vi "digitally_ros_joystick.vi"() -> ()   [LabVIEW 2019]
uses:
  <vilib>/addons/eal4LabVIEW/ApiLib/Connection control/ealApiConnect_string.vi
  <vilib>/Utility/inputDevices.llb/joystickAcquire.vi
  <vilib>/Utility/inputDevices.llb/closeJoystick.vi
  <vilib>/addons/eal4LabVIEW/eal4LabVIEW.lvlib
panel:
  out "I value":i32
  out "Y axis 2":i32
  out "Y axis":i32
  out "X axis":i32
  out "error out":errorcluster
  out "Is joystick used?":bool
  out "Is manual control on?":bool
  out "RPM 3 Joystick":dbl
  out "RPM 1 Joystick":dbl
  out "RPM 2 Joystick":dbl
  out "Is joystick used?":bool[](array[boolean])
  in  "Activate manual control":bool
  out "Is the PID fnished?":bool[](array[boolean])
  out "In Range? (1)":bool
  out "In Range? (2)":bool
  out "In Range? (3)":bool
  in  "condition 6":i32(ring) items=["AXIS_CONDITION_ACTIVE"=0, "AXIS_CONDITION_PARKING"=1, "AXIS_CONDITION_DEACTIVATED"=2, "AXIS_CONDITION_ACTIVE_DECOUPLED"=4, "AXIS_CONDITION_PARKING_DECOUPLED"=5, "AXIS_CONDITION_DEACTIVATED_DECOUPLED"=6, "AXIS_CONDITION_ACTIVE_PARAMETERIZATION"=8, "AXIS_CONDITION_PARKING_PARAMETERIZATION"=9, "AXIS_CONDITION_DEACTIVATED_PARAMETERIZATION"=10, "AXIS_CONDITION_ACTIVE_DECOUPLED_PARAMETERIZATION"=12, "AXIS_CONDITION_PARKING_DECOUPLED_PARAMETERIZATION"=13, "AXIS_CONDITION_DEACTIVATED_DECOUPLED_PARAMETERIZATION"=14]
  in  "slave index 6":i32
  in  "condition 5":i32(ring) items=["AXIS_CONDITION_ACTIVE"=0, "AXIS_CONDITION_PARKING"=1, "AXIS_CONDITION_DEACTIVATED"=2, "AXIS_CONDITION_ACTIVE_DECOUPLED"=4, "AXIS_CONDITION_PARKING_DECOUPLED"=5, "AXIS_CONDITION_DEACTIVATED_DECOUPLED"=6, "AXIS_CONDITION_ACTIVE_PARAMETERIZATION"=8, "AXIS_CONDITION_PARKING_PARAMETERIZATION"=9, "AXIS_CONDITION_DEACTIVATED_PARAMETERIZATION"=10, "AXIS_CONDITION_ACTIVE_DECOUPLED_PARAMETERIZATION"=12, "AXIS_CONDITION_PARKING_DECOUPLED_PARAMETERIZATION"=13, "AXIS_CONDITION_DEACTIVATED_DECOUPLED_PARAMETERIZATION"=14]
  in  "slave index 5":i32
  in  "condition 4":i32(ring) items=["AXIS_CONDITION_ACTIVE"=0, "AXIS_CONDITION_PARKING"=1, "AXIS_CONDITION_DEACTIVATED"=2, "AXIS_CONDITION_ACTIVE_DECOUPLED"=4, "AXIS_CONDITION_PARKING_DECOUPLED"=5, "AXIS_CONDITION_DEACTIVATED_DECOUPLED"=6, "AXIS_CONDITION_ACTIVE_PARAMETERIZATION"=8, "AXIS_CONDITION_PARKING_PARAMETERIZATION"=9, "AXIS_CONDITION_DEACTIVATED_PARAMETERIZATION"=10, "AXIS_CONDITION_ACTIVE_DECOUPLED_PARAMETERIZATION"=12, "AXIS_CONDITION_PARKING_DECOUPLED_PARAMETERIZATION"=13, "AXIS_CONDITION_DEACTIVATED_DECOUPLED_PARAMETERIZATION"=14]
  in  "slave index 4":i32
  out "RPM 1 ROS":dbl
  out "RPM 2 ROS":dbl
  out "RPM 3 ROS":dbl
  in  "stop":bool
  out "Return value":dbl[](array[numeric])
  out "Iteration counter":i32
  # "ROS Control"
  # "Joystick Control"
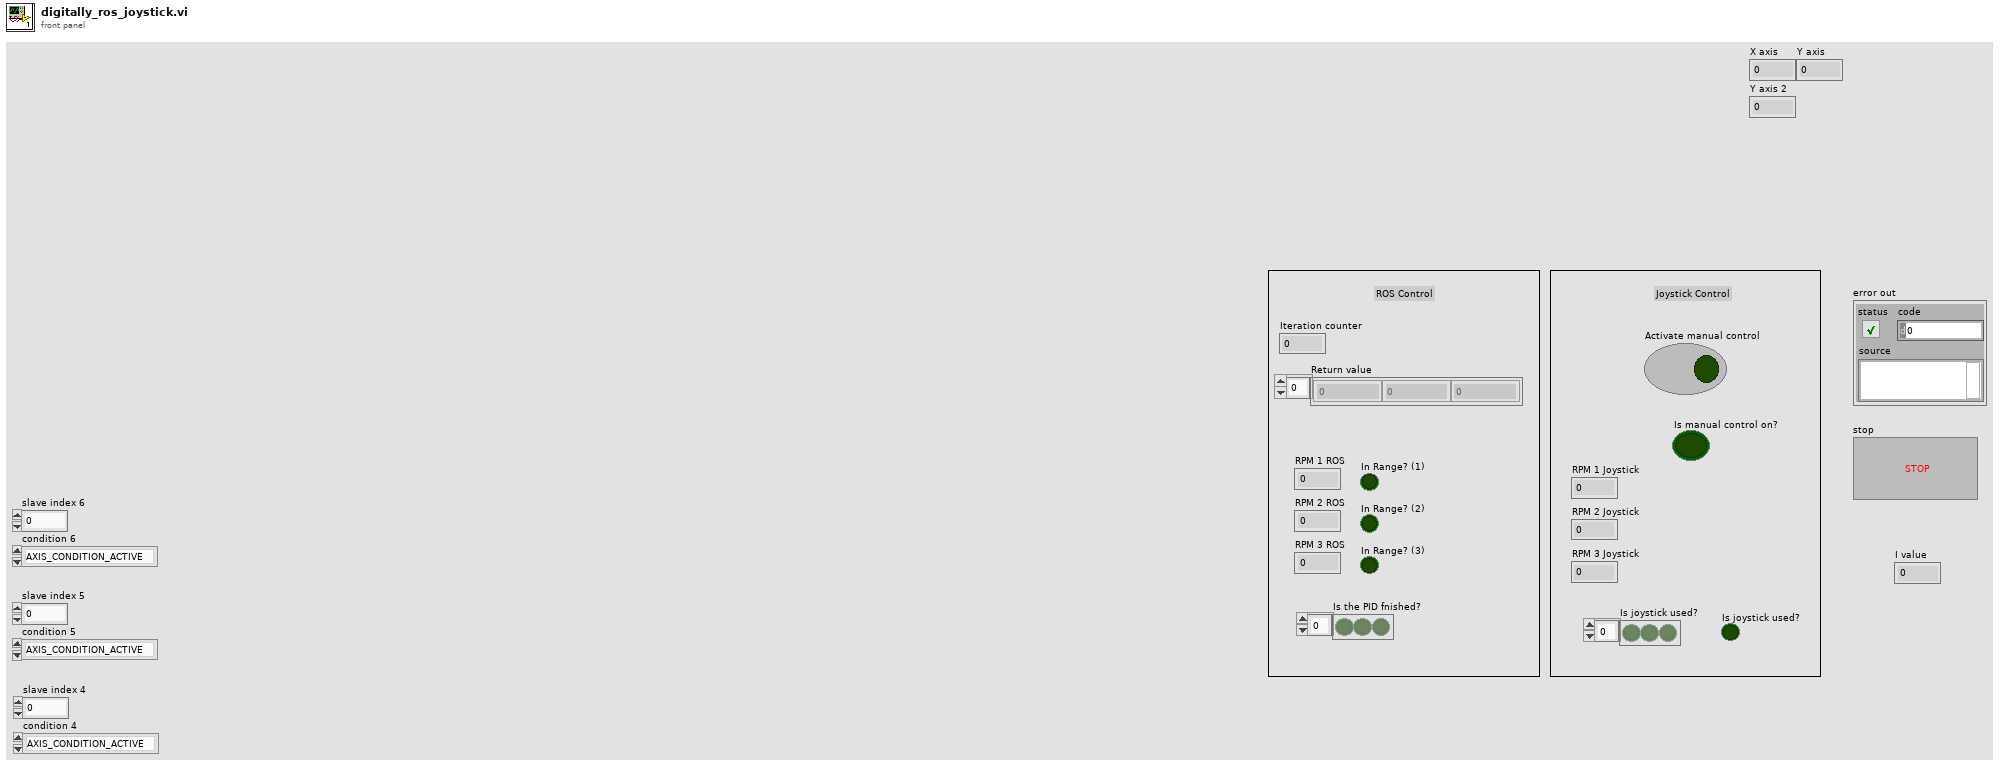
[diagram p1: front panel]
types:
  T1 = cluster{"Velocity":dbl, "Acceleration":dbl, "Deceleration":dbl, "Jerk":dbl}
  T2 = cluster{"X axis":i32, "Y axis":i32, "Z axis":i32, "X axis rotation":i32, "Y axis rotation":i32, "Z axis rotation":i32, "U axis":i32, "V axis":i32}
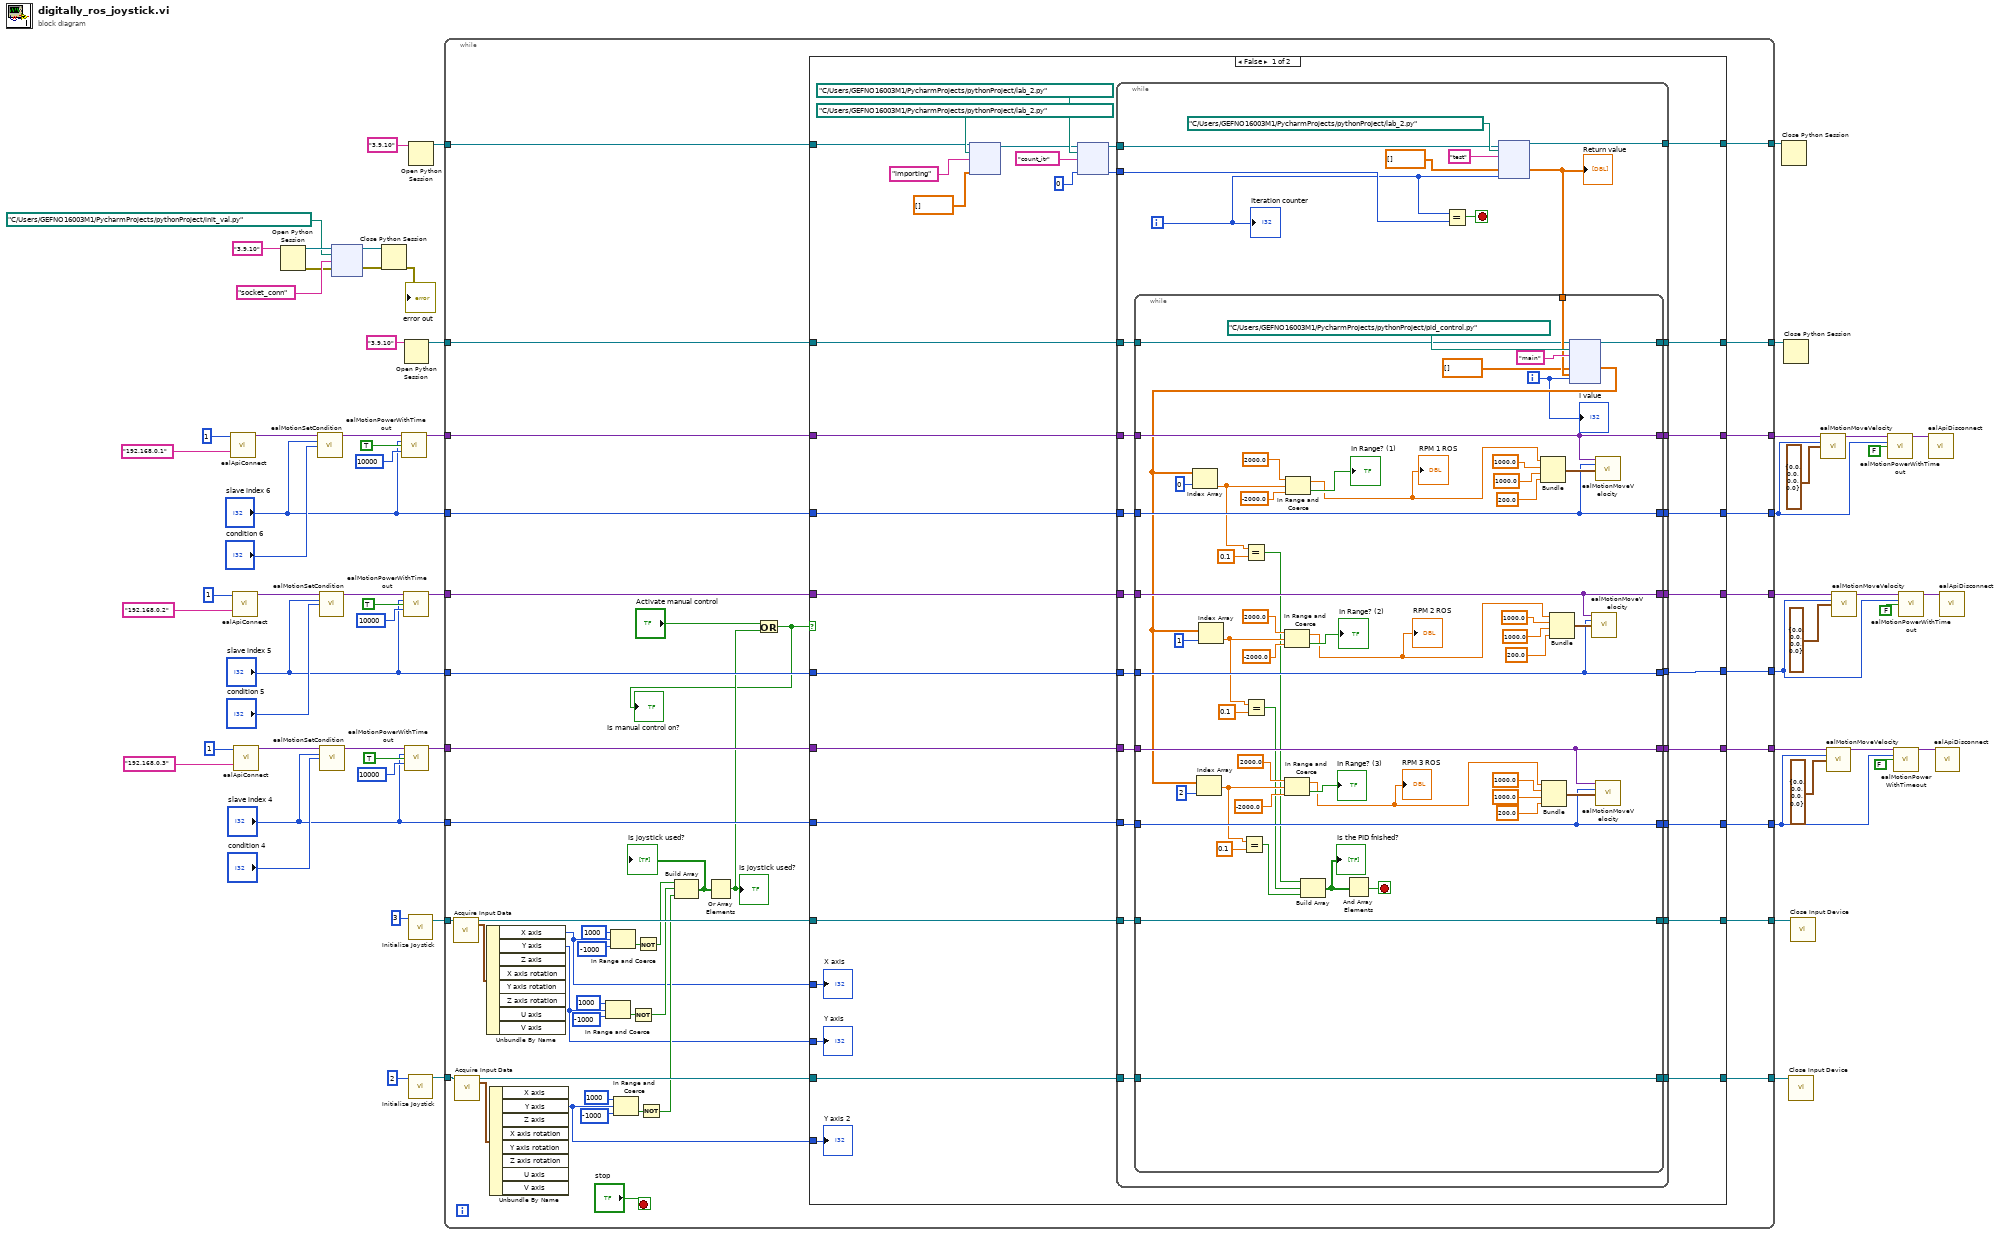
[diagram p0: block diagram]
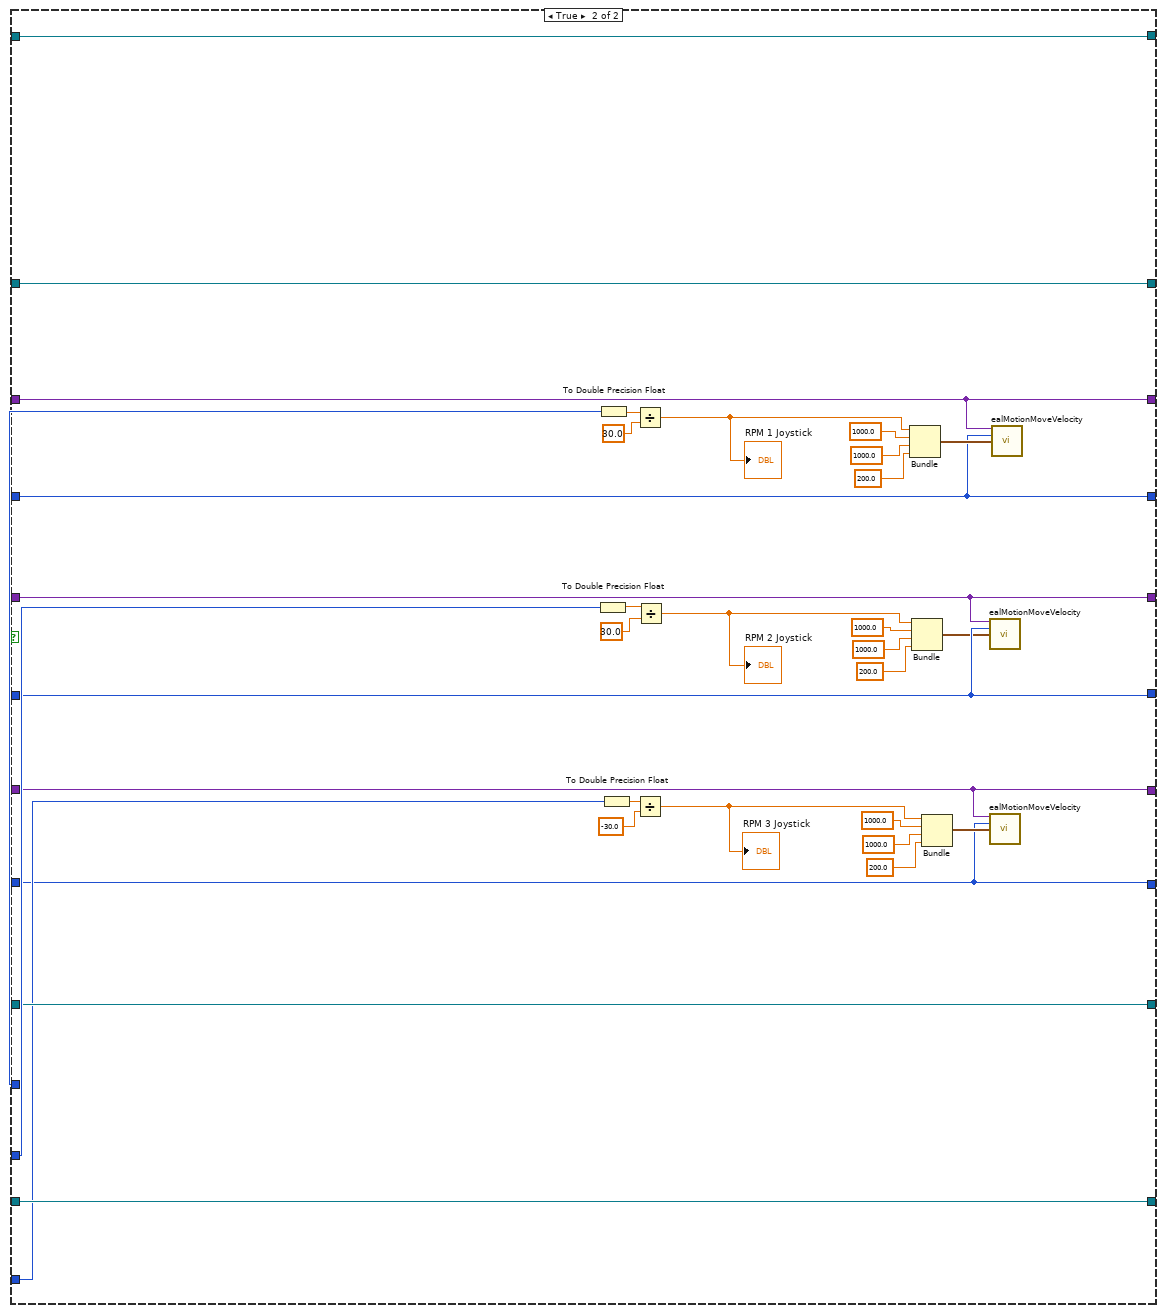
[diagram p2: hidden frame]
diagram:
  n1 = call-poly <vilib>:"ealApiConnect.vi"("maximum no of axes"=1, "ip address"="192.168.0.1") -> ("connection out"=w37:variant)  [unwired: 12 in, 1 out]
  n2 = call-poly <vilib>:"ealApiConnect.vi"("maximum no of axes"=1, "ip address"="192.168.0.2") -> ("connection out"=w44:variant)  [unwired: 12 in, 1 out]
  n3 = call-poly <vilib>:"ealApiConnect.vi"("maximum no of axes"=1, "ip address"="192.168.0.3") -> ("connection out"=w51:variant)  [unwired: 12 in, 1 out]
  n4 = Open Python Session(python version="3.9.10" ("Python version")) -> (session out=w7:refnum<k35>, error out=w3:errorcluster)  [unwired: 2 in]
  n5 = call <vilib>:"ealMotionSetCondition.vi"("connection in"=w37, "slave index"="slave index 6", "condition"="condition 6") -> ("connection out"=w36:variant)  [unwired: 11 in, 1 out]
  n6 = call <vilib>:"ealMotionSetCondition.vi"("connection in"=w44, "slave index"="slave index 5", "condition"="condition 5") -> ("connection out"=w43:variant)  [unwired: 11 in, 1 out]
  n7 = call <vilib>:"ealMotionSetCondition.vi"("connection in"=w51, "slave index"="slave index 4", "condition"="condition 4") -> ("connection out"=w50:variant)  [unwired: 11 in, 1 out]
  n8 = node(w7, path "C:/Users/GEFNO16003M1/PycharmProjects/pythonProject/init_val.py" ("module path"), "socket_conn" ("function name"), w3) -> (w6:refnum<k35>, w2:errorcluster)  [unwired: 2 in, 2 out]
  n9 = Close Python Session(session in=w6, error in=w2) -> (11:→"error out":errorcluster)
  n10 = call <vilib>:"ealMotionPowerWithTimeout.vi"("connection in"=w36, "slave index"="slave index 6", "value"=TRUE, "timeout"=10000) -> ("connection out"=w32:variant)  [unwired: 10 in, 1 out]
  n11 = call <vilib>:"ealMotionPowerWithTimeout.vi"("connection in"=w43, "slave index"="slave index 5", "value"=TRUE, "timeout"=10000) -> ("connection out"=w31:variant)  [unwired: 10 in, 1 out]
  n12 = Open Python Session(python version="3.9.10" ("Python version")) -> (session out=w18:refnum<k35>)  [unwired: 2 in, 1 out]
  n13 = call <vilib>:"ealMotionPowerWithTimeout.vi"("connection in"=w50, "slave index"="slave index 4", "value"=TRUE, "timeout"=10000) -> ("connection out"=w30:variant)  [unwired: 10 in, 1 out]
  n14 = call <vilib>:"Initialize Joystick.vi"("device index"=3) -> ("device ID"=w12:refnum<k1>)  [unwired: 9 in, 1 out]
  n15 = call <vilib>:"Initialize Joystick.vi"("device index"=2) -> ("device ID"=w11:refnum<k1>)  [unwired: 9 in, 1 out]
  n16 = Open Python Session(python version="3.9.10" ("Python version")) -> (session out=w21:refnum<k35>)  [unwired: 2 in, 1 out]
  n17 = while {
    tunnel: w32 -> [w108]
    tunnel: w31 -> [w107]
    tunnel: w30 -> [w106]
    tunnel: [w84] -> w29
    tunnel: [w105] -> w28
    tunnel: "slave index 6" -> [w104]
    tunnel: "slave index 5" -> [w103]
    tunnel: [w102] -> w25
    tunnel: [w96] -> w24
    tunnel: "slave index 4" -> [w101]
    tunnel: w21 -> [w100]
    tunnel: [w99] -> w20
    tunnel: w18 -> [w98]
    tunnel: [w85] -> w17
    tunnel: [w97] -> w16
    tunnel: [w95] -> w15
    tunnel: w12 -> [w92]
    tunnel: w11 -> [w89]
    tunnel: [w94] -> w10
    tunnel: [w93] -> w9
    stop <- "stop" stop-if-true
    n18 = call-poly <vilib>:"Acquire Input Data.vi"("device ID"=w92) -> ("device ID"=w91:refnum<k1>, "axis info"=w90:T2)  [unwired: 14 in, 3 out]
    n19 = call-poly <vilib>:"Acquire Input Data.vi"("device ID"=w89) -> ("device ID"=w88:refnum<k1>, "axis info"=w87:T2)  [unwired: 14 in, 3 out]
    n20 = Unbundle By Name(w90) -> ("X axis"=w68:i32, "Y axis"=w75:i32)  [unwired: 6 out]
    n21 = Unbundle By Name(w87) -> ("Y axis"=w82:i32)  [unwired: 7 out]
    n22 = In Range and Coerce(upper limit=1000, x=w75, lower limit=-1000) -> (In Range?=w77:bool)  [unwired: 1 out]
    n23 = In Range and Coerce(upper limit=1000, x=w68, lower limit=-1000) -> (In Range?=w72:bool)  [unwired: 1 out]
    n24 = In Range and Coerce(upper limit=1000, x=w82, lower limit=-1000) -> (In Range?=w81:bool)  [unwired: 1 out]
    n25 = Not(x=w77) -> (.not. x?=w73:bool)
    n26 = Not(x=w72) -> (.not. x?=w69:bool)
    n27 = Not(x=w81) -> (.not. x?=w80:bool)
    n28 = Build Array(w69, w73, w80) -> (w83:bool[])
    "Is joystick used?" <- w83
    n29 = Or Array Elements(Boolean array=w83) -> (logical OR=w67:bool)
    "Is joystick used?" <- w67
    n30 = Or(x="Activate manual control", y=w67) -> (x .or. y?=w66:bool)
    "Is manual control on?" <- w66
    n31 = case shown="False" w66 {
      tunnel: w108 -> [w132 w234]
      tunnel: w107 -> [w131 w231]
      tunnel: w106 -> [w130 w225]
      tunnel: [w129 w230] -> w105
      tunnel: w104 -> [w128 w230]
      tunnel: w103 -> [w127 w229]
      tunnel: [w126 w229] -> w102
      tunnel: w101 -> [w125 w223]
      tunnel: w100 -> [w124 w256]
      tunnel: [w123 w256] -> w99
      tunnel: w98 -> [w122 w255]
      tunnel: [w121 w223] -> w97
      tunnel: [w120 w231] -> w96
      tunnel: [w119 w255] -> w95
      tunnel: [w118 w246] -> w94
      tunnel: [w117 w245] -> w93
      tunnel: w91 -> [w116 w246]
      tunnel: w88 -> [w115 w245]
      tunnel: [w114 w225] -> w85
      tunnel: w75 -> [w111 w248]
      tunnel: w68 -> [w112 w247]
      tunnel: [w113 w234] -> w84
      tunnel: w82 -> [w110 w244]
      frame False {
        n32 = node(w124, path "C:/Users/GEFNO16003M1/PycharmProjects/pythonProject/lab_2.py" ("module path"), "importing" ("function name"), dbl[] []) -> (w136:refnum<k35>)  [unwired: 2 in, 3 out]
        n33 = node(w136, path "C:/Users/GEFNO16003M1/PycharmProjects/pythonProject/lab_2.py" ("module path"), "count_itr" ("function name"), 0) -> (w135:refnum<k35>, w133:i32)  [unwired: 1 in, 3 out]
        n34 = while {
          tunnel: [w162] -> w123
          tunnel: w135 -> [w165]
          tunnel: w133 -> [w163]
          tunnel: w132 -> [w160]
          tunnel: w131 -> [w149]
          tunnel: w130 -> [w159]
          tunnel: [w151] -> w113
          tunnel: [w152] -> w129
          tunnel: w128 -> [w150]
          tunnel: w127 -> [w148]
          tunnel: [w153] -> w126
          tunnel: w125 -> [w155]
          tunnel: w122 -> [w147]
          tunnel: [w157] -> w114
          tunnel: [w156] -> w121
          tunnel: [w154] -> w120
          tunnel: [w146] -> w119
          tunnel: w116 -> [w145]
          tunnel: w115 -> [w144]
          tunnel: [w143] -> w118
          tunnel: [w142] -> w117
          i -> [w158]
          stop <- w166 stop-if-true
          n35 = Equal?(x=w158, y=w163) -> (x = y?=w166:bool)
          n36 = node(w165, path "C:/Users/GEFNO16003M1/PycharmProjects/pythonProject/lab_2.py" ("module path"), "test" ("function name"), dbl[] [], w158) -> (w162:refnum<k35>, w161:dbl[])  [unwired: 2 in, 3 out]
          "Return value" <- w161
          n37 = while {
            tunnel: w161 -> [w220]
            tunnel: w160 -> [w192]
            tunnel: w159 -> [w194]
            tunnel: [w194] -> w157
            tunnel: [w193] -> w156
            tunnel: w155 -> [w193]
            tunnel: [w190] -> w154
            tunnel: [w189] -> w153
            tunnel: [w191] -> w152
            tunnel: [w192] -> w151
            tunnel: w150 -> [w191]
            tunnel: w149 -> [w190]
            tunnel: w148 -> [w189]
            tunnel: w147 -> [w188]
            tunnel: [w187] -> w146
            tunnel: w145 -> [w171]
            tunnel: w144 -> [w170]
            tunnel: [w171] -> w143
            tunnel: [w170] -> w142
            i -> [w169]
            stop <- w185 stop-if-true
            n38 = node(w188, path "C:/Users/GEFNO16003M1/PycharmProjects/pythonProject/pid_control.py" ("module path"), "main" ("function name"), dbl[] [], w220, w169) -> (w187:refnum<k35>, w186:dbl[])  [unwired: 3 in, 3 out]
            n39 = Index Array(array=w186, index=0) -> (element=w181:dbl)
            n40 = Index Array(array=w186, index=2) -> (element=w179:dbl)
            n41 = Index Array(array=w186, index=1) -> (element=w180:dbl)
            n42 = Equal?(x=w179, y=0.1) -> (x = y?=w176:bool)
            n43 = Equal?(x=w181, y=0.1) -> (x = y?=w178:bool)
            n44 = Equal?(x=w180, y=0.1) -> (x = y?=w177:bool)
            n45 = In Range and Coerce(upper limit=2000.0, x=w180, lower limit=-2000.0) -> (coerced(x)=w173:dbl, In Range?=→"In Range? (2)":bool)
            "RPM 2 ROS" <- w173
            n46 = In Range and Coerce(upper limit=2000.0, x=w179, lower limit=-2000.0) -> (coerced(x)=w172:dbl, In Range?=→"In Range? (3)":bool)
            "RPM 3 ROS" <- w172
            n47 = In Range and Coerce(upper limit=2000.0, x=w181, lower limit=-2000.0) -> (coerced(x)=w174:dbl, In Range?=→"In Range? (1)":bool)
            "RPM 1 ROS" <- w174
            n48 = Build Array(w178, w177, w176) -> (w175:bool[])
            "Is the PID fnished?" <- w175
            n49 = And Array Elements(Boolean array=w175) -> (logical AND=w185:bool)
            n50 = Bundle("upper limit"=w174, 1000.0, 1000.0, 200.0) -> (w204:cluster{"upper limit":dbl, dbl, dbl, dbl})  [unwired: 1 in]
            n51 = Bundle("upper limit"=w172, 1000.0, 1000.0, 200.0) -> (w214:cluster{"upper limit":dbl, dbl, dbl, dbl})  [unwired: 1 in]
            n52 = Bundle("upper limit"=w173, 1000.0, 1000.0, 200.0) -> (w209:cluster{"upper limit":dbl, dbl, dbl, dbl})  [unwired: 1 in]
            n53 = call <vilib>:"ealMotionMoveVelocity.vi"("connection in"=w190, "slave index"=w189, "parameters set"=w209) -> ()  [unwired: 11 in, 2 out]
            n54 = call <vilib>:"ealMotionMoveVelocity.vi"("connection in"=w192, "slave index"=w191, "parameters set"=w204) -> ()  [unwired: 11 in, 2 out]
            n55 = call <vilib>:"ealMotionMoveVelocity.vi"("connection in"=w194, "slave index"=w193, "parameters set"=w214) -> ()  [unwired: 11 in, 2 out]
            "I value" <- w169
          }
          "Iteration counter" <- w158
        }
        "X axis" <- w112
        "Y axis" <- w111
        "Y axis 2" <- w110
      }
      frame True {
        n56 = To Double Precision Float(number=w248) -> (double precision float=w252:dbl)
        n57 = To Double Precision Float(number=w247) -> (double precision float=w253:dbl)
        n58 = To Double Precision Float(number=w244) -> (double precision float=w254:dbl)
        n59 = Divide(x=w253, y=30.0) -> (x/y=w233:dbl)
        "RPM 1 Joystick" <- w233
        n60 = Divide(x=w254, y=-30.0) -> (x/y=w224:dbl)
        "RPM 3 Joystick" <- w224
        n61 = Divide(x=w252, y=30.0) -> (x/y=w227:dbl)
        "RPM 2 Joystick" <- w227
        n62 = Bundle(w233, 1000.0, 1000.0, 200.0) -> (w232:cluster{dbl, dbl, dbl, dbl})  [unwired: 1 in]
        n63 = Bundle(w227, 1000.0, 1000.0, 200.0) -> (w228:cluster{dbl, dbl, dbl, dbl})  [unwired: 1 in]
        n64 = Bundle(w224, 1000.0, 1000.0, 200.0) -> (w226:cluster{dbl, dbl, dbl, dbl})  [unwired: 1 in]
        n65 = call <vilib>:"ealMotionMoveVelocity.vi"("connection in"=w231, "slave index"=w229, "parameters set"=w228) -> ()  [unwired: 11 in, 2 out]
        n66 = call <vilib>:"ealMotionMoveVelocity.vi"("connection in"=w225, "slave index"=w223, "parameters set"=w226) -> ()  [unwired: 11 in, 2 out]
        n67 = call <vilib>:"ealMotionMoveVelocity.vi"("connection in"=w234, "slave index"=w230, "parameters set"=w232) -> ()  [unwired: 11 in, 2 out]
      }
    }
  }
  n68 = Close Python Session(session in=w20) -> ()  [unwired: 1 in, 1 out]
  n69 = Close Python Session(session in=w15) -> ()  [unwired: 1 in, 1 out]
  n70 = call-poly <vilib>:"Close Input Device.vi"("device ID"=w9) -> ()  [unwired: 9 in, 1 out]
  n71 = call-poly <vilib>:"Close Input Device.vi"("device ID"=w10) -> ()  [unwired: 9 in, 1 out]
  n72 = call <vilib>:"ealMotionMoveVelocity.vi"("connection in"=w29, "slave index"=w28, "parameters set"=T1 {"Velocity"=0.0, "Acceleration"=0.0, "Deceleration"=0.0, "Jerk"=0.0}) -> ("connection out"=w56:variant)  [unwired: 11 in, 1 out]
  n73 = call <vilib>:"ealMotionMoveVelocity.vi"("connection in"=w17, "slave index"=w16, "parameters set"=T1 {"Velocity"=0.0, "Acceleration"=0.0, "Deceleration"=0.0, "Jerk"=0.0}) -> ("connection out"=w64:variant)  [unwired: 11 in, 1 out]
  n74 = call <vilib>:"ealMotionMoveVelocity.vi"("connection in"=w24, "slave index"=w25, "parameters set"=T1 {"Velocity"=0.0, "Acceleration"=0.0, "Deceleration"=0.0, "Jerk"=0.0}) -> ("connection out"=w60:variant)  [unwired: 11 in, 1 out]
  n75 = call <vilib>:"ealMotionPowerWithTimeout.vi"("connection in"=w56, "slave index"=w28, "value"=FALSE) -> ("connection out"=w57:variant)  [unwired: 11 in, 1 out]
  n76 = call <vilib>:"ealMotionPowerWithTimeout.vi"("connection in"=w64, "slave index"=w16, "value"=FALSE) -> ("connection out"=w65:variant)  [unwired: 11 in, 1 out]
  n77 = call <vilib>:"ealMotionPowerWithTimeout.vi"("connection in"=w60, "slave index"=w25, "value"=FALSE) -> ("connection out"=w61:variant)  [unwired: 11 in, 1 out]
  n78 = call <vilib>:"ealApiDisconnect.vi"("connection in"=w57) -> ()  [unwired: 14 in, 1 out]
  n79 = call <vilib>:"ealApiDisconnect.vi"("connection in"=w65) -> ()  [unwired: 14 in, 1 out]
  n80 = call <vilib>:"ealApiDisconnect.vi"("connection in"=w61) -> ()  [unwired: 14 in, 1 out]
